vi "Read Section Name.vi"(8 "error in (no error)":errorcluster, 11 "Configuration File in":refnum<class "Configuration File.lvclass">) -> (0 "error out":errorcluster, 3 "Configuration File out":refnum<class "Configuration File.lvclass">)   [LabVIEW 2020, in "Configuration File.lvclass"]
uses:
  Configuration File.lvclass
  Process/Process.lvclass
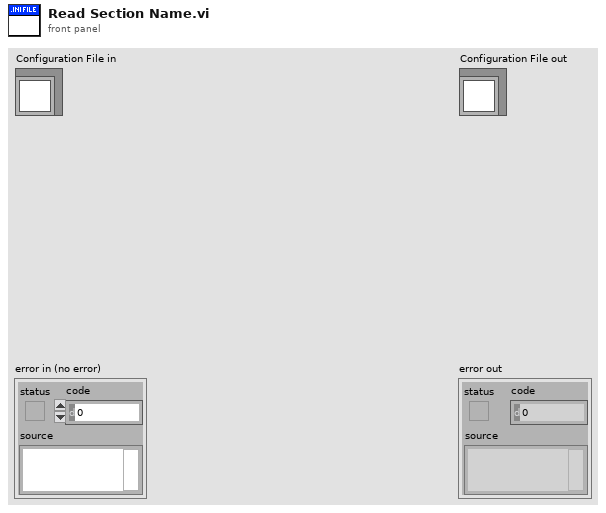
[diagram p1: front panel]
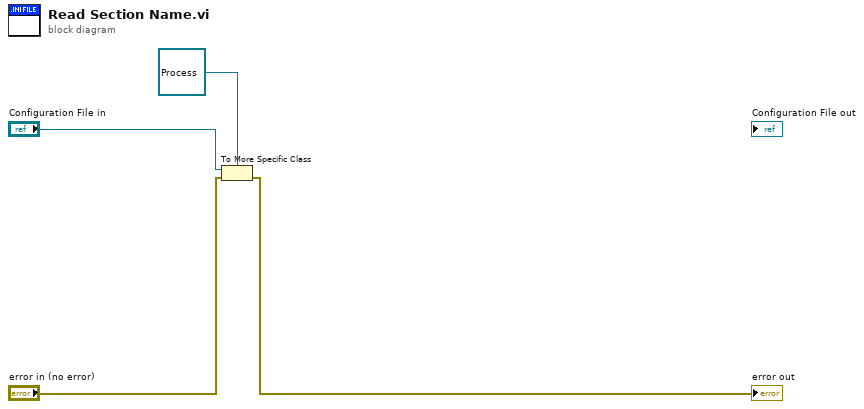
[diagram p0: block diagram]
diagram:
  n1 = To More Specific Class(target class=refnum<class "Process.lvclass"> refnum ("Process.lvclass"), reference="Configuration File in", error in="error in (no error)") -> (error out=→"error out":errorcluster)  [unwired: 1 out]
